vi "procesSiMAGE.vi"(0 "Cam Cluster out":T6={"incident ANGLE COMPENSATION"=[], "field of view /pixel"=0.0, "dp/B [MeV/C/B]"=[], "charge compensation"=[], "Momentum [MeV/C]"=[], "B [T]"=1.0, "energyDependence Input"=[], "pixel angle (y)"=[], "dp [MeV/C/] "=[], "angle 2Dfor spectrumj"=[], "dp [MeV/C] 2D"=[], "charge compensation 2D"=[], "Screen&Camera 2"={"Screen Orientation"="Regular", "Screen angle"="Flat", "Lens"=enum."FL1-f8x08", "Calibration (mm/pix)"=1.0}, "ROI info"={"npix-X"=0, "npix-Y"=0, "Left [pix]"=0.0, "Top [pix]"=0.0}, "Y 2D full angle"=[]}, 1 "Image":T2, 2 "empty image":bool, 5 "CamSettings.Cam 0":T3={"position"=0.0, "Field of view"=0.0, "start"=0.0, "end"=0.0, "center"=0.0, "Lens"=enum."FL1-f8x08", "Forward"=enum."off", "Spec_Calib_file 2"=path "Y:/100TWdata/ESMCalib/datFwd.txt", "map"=path "Y:/100TWdata/ESMCalib/mapFwd.txt", "y size"=0}, 12 "B [T]":dbl) -> (4 "Cam Cluster out 2":T6={"incident ANGLE COMPENSATION"=[], "field of view /pixel"=0.0, "dp/B [MeV/C/B]"=[], "charge compensation"=[], "Momentum [MeV/C]"=[], "B [T]"=1.0, "energyDependence Input"=[], "pixel angle (y)"=[], "dp [MeV/C/] "=[], "angle 2Dfor spectrumj"=[], "dp [MeV/C] 2D"=[], "charge compensation 2D"=[], "Screen&Camera 2"={"Screen Orientation"="Regular", "Screen angle"="Flat", "Lens"=enum."FL1-f8x08", "Calibration (mm/pix)"=1.0}, "ROI info"={"npix-X"=0, "npix-Y"=0, "Left [pix]"=0.0, "Top [pix]"=0.0}, "Y 2D full angle"=[]}, 6 "Sum Y":cluster{"Ramp Pattern":dbl[], dbl[]}, 8 "spec cluster":cluster{"dp [MeV/C]":dbl[], dbl[]}(graph), 10 "z":dbl[][](array[numeric]), 14 "time":u32)   [LabVIEW 2011]
uses:
  calib_Sub_Typdef.ctl
  ScreenCam2_TypDEf.ctl
  CamAndObj_TypDEf.ctl
  ROIInfo_TypDef.ctl
  CamSettingSUB_TypDEf.ctl
  OnOffTypeDef.ctl
  IMAQ Image.ctl
panel:
  out "x*y":dbl[][](array[numeric])
  out "time 2":u32
  out "spec cluster 2":T1(graph)
  out "Momentum [MeV/C]":dbl[](array[numeric])
  out "Boolean":bool
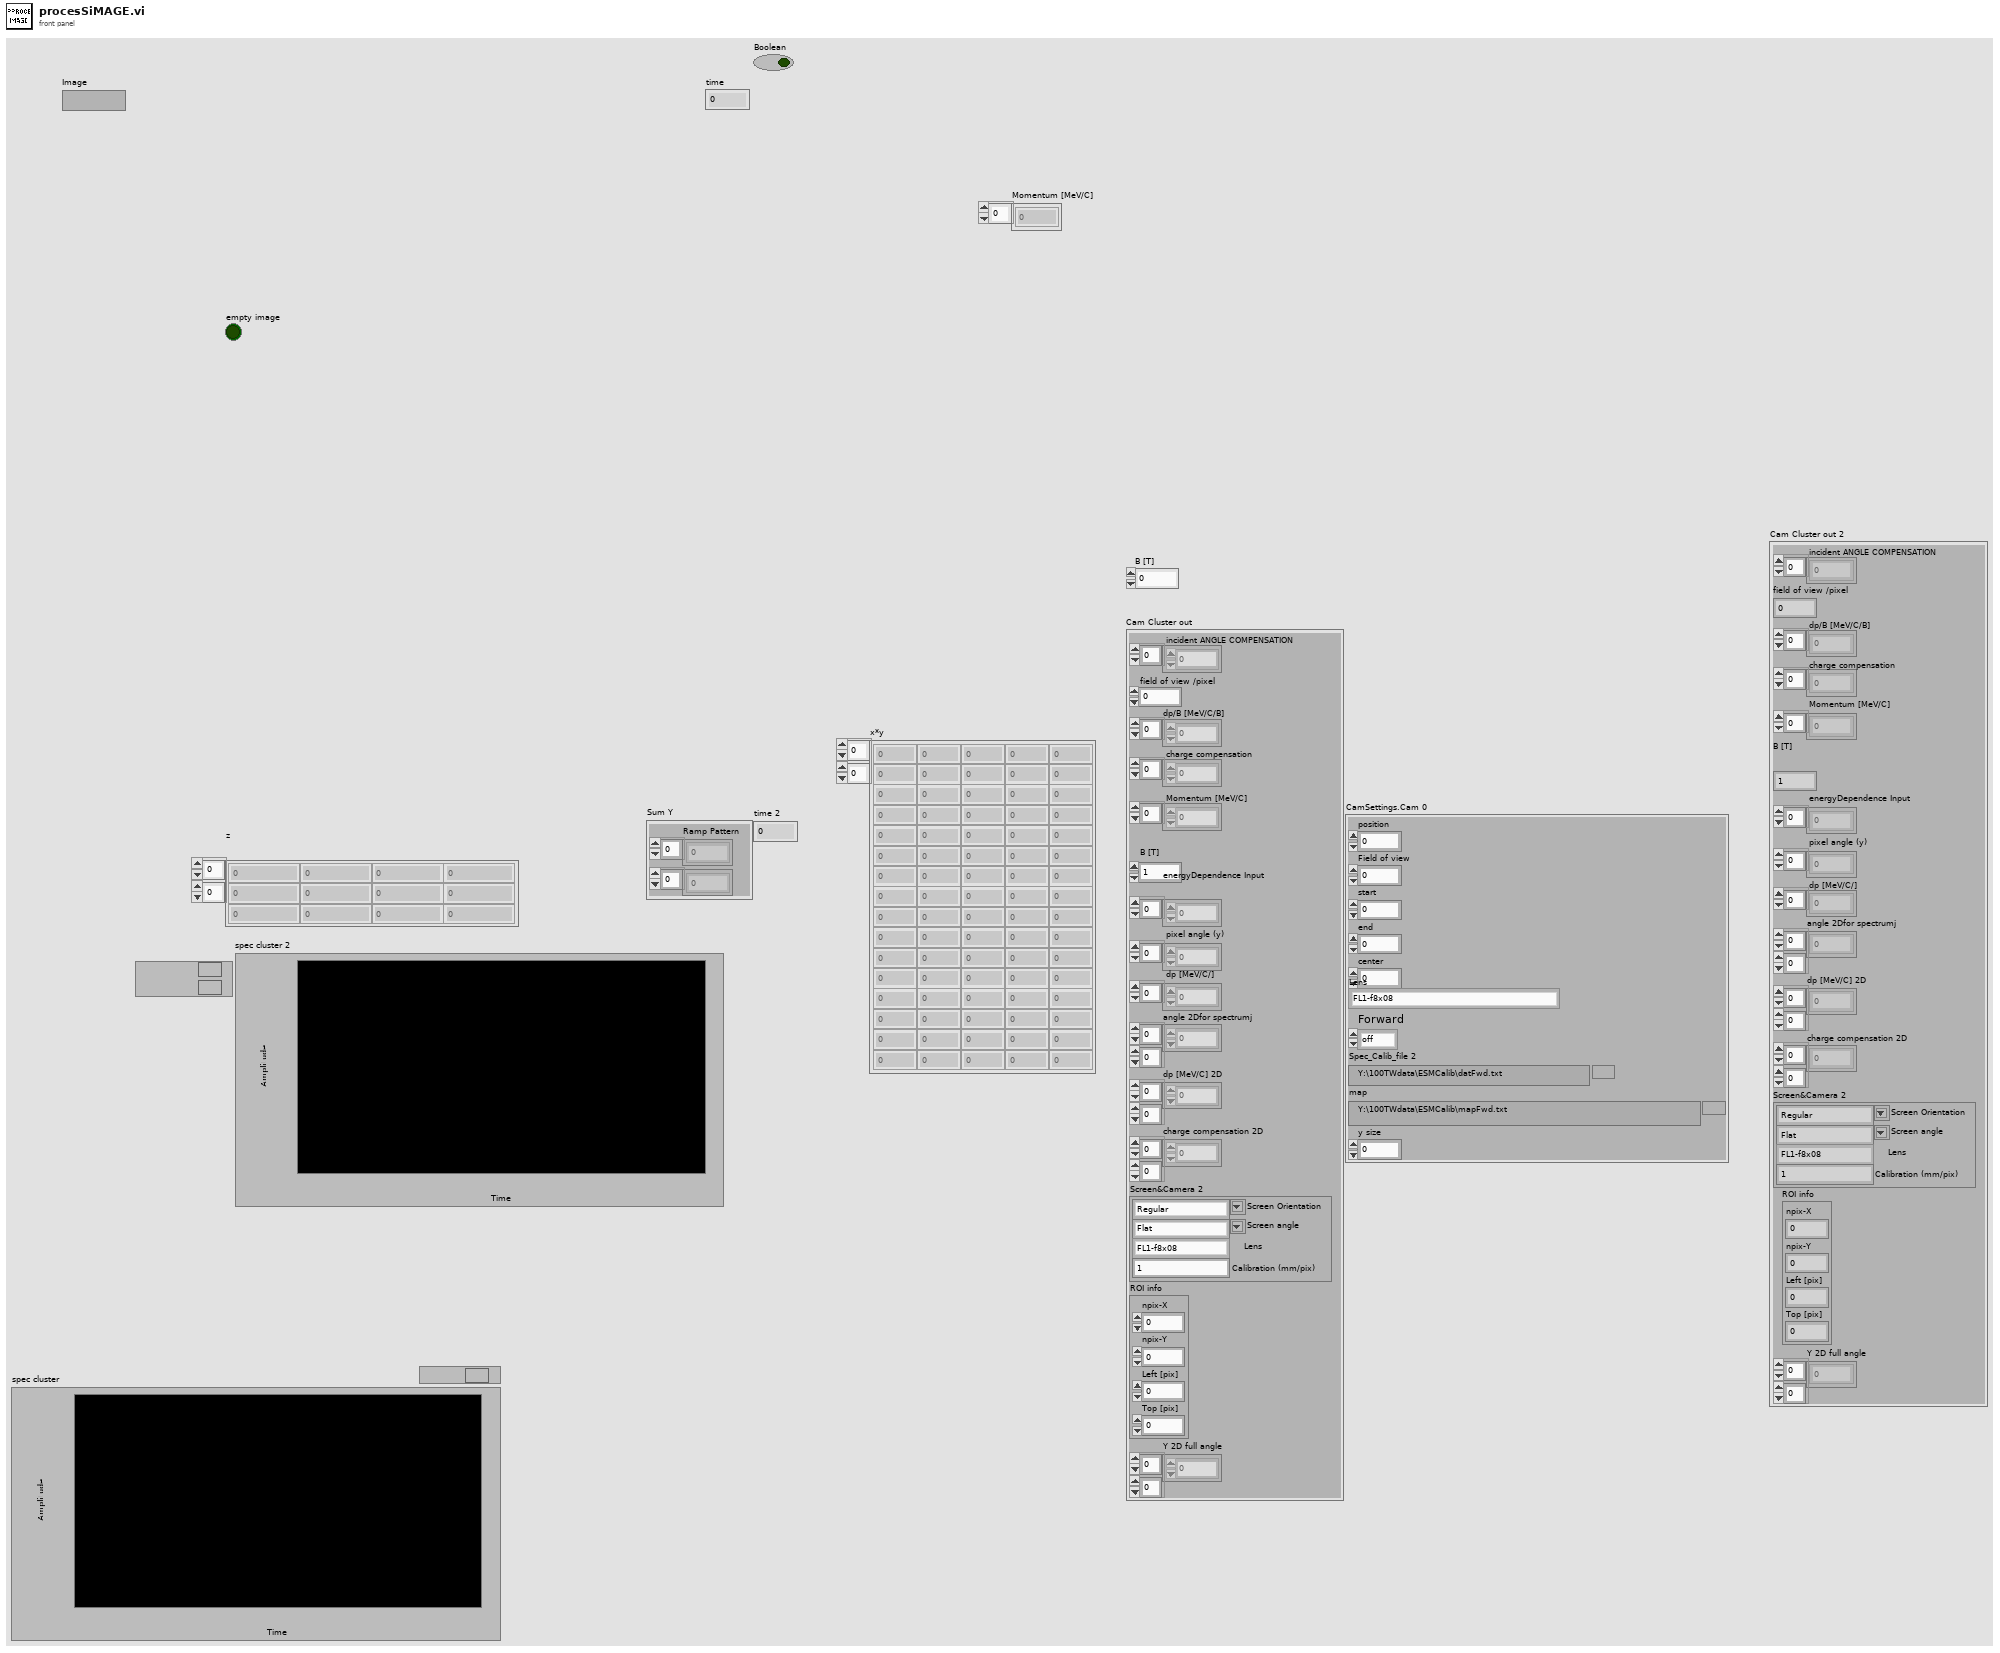
[diagram p1: front panel]
types:
  T1 = cluster{"Momentum [MeV/C]":dbl[], "Sum X (spectra)":dbl[]}[]
  T2 = typedef "IMAQ Image.ctl" = refnum<image>
  T3 = typedef "CamSettingSUB_TypDEf.ctl" = cluster{"position":dbl, "Field of view":dbl, "start":dbl, "end":dbl, "center":dbl, "Lens":T4, "Forward":T5, "Spec_Calib_file 2":path, "map":path, "y size":i32}
  T4 = typedef "CamAndObj_TypDEf.ctl" = enum16{"FL1-f8x08", "FL1-f8x06", "FL1-f8", "ch300-f50", "FL2G-f8", "FL3M14-f8", "FL3M14-f8x08", "FL3M14-f8x08(2x2)"}
  T5 = typedef "OnOffTypeDef.ctl" = enum16{"off", "on"}
  T6 = typedef "calib_Sub_Typdef.ctl" = cluster{"incident ANGLE COMPENSATION":dbl[], "field of view /pixel":dbl, "dp/B [MeV/C/B]":dbl[], "charge compensation":dbl[], "Momentum [MeV/C]":dbl[], "B [T]":dbl, "energyDependence Input":dbl[], "pixel angle (y)":dbl[], "dp [MeV/C/] ":dbl[], "angle 2Dfor spectrumj":dbl[][], "dp [MeV/C] 2D":dbl[][], "charge compensation 2D":dbl[][], "Screen&Camera 2":T7, "ROI info":T8, "Y 2D full angle":dbl[][]}
  T7 = typedef "ScreenCam2_TypDEf.ctl" = cluster{"Screen Orientation":string, "Screen angle":string, "Lens":T4, "Calibration (mm/pix)":dbl}
  T8 = typedef "ROIInfo_TypDef.ctl" = cluster{"npix-X":i32, "npix-Y":i32, "Left [pix]":dbl, "Top [pix]":dbl}
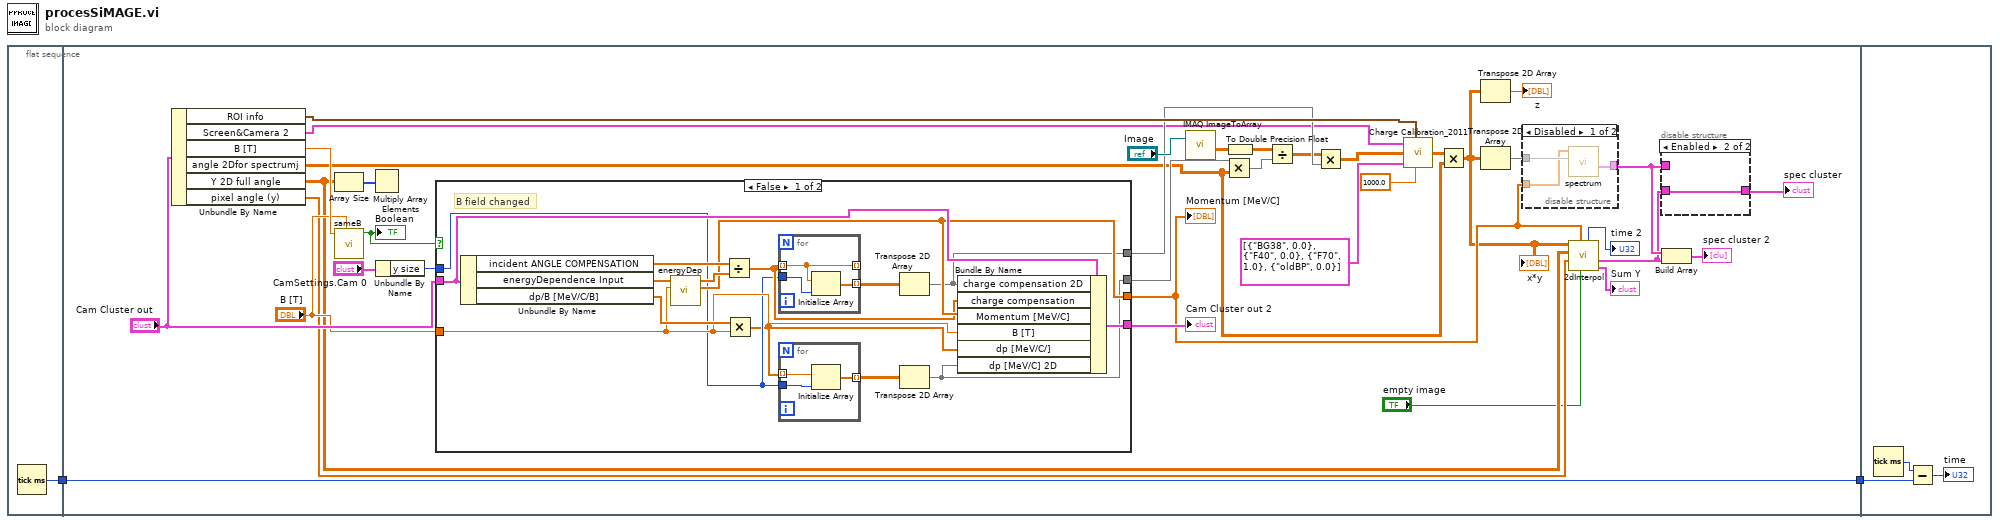
[diagram p0: block diagram]
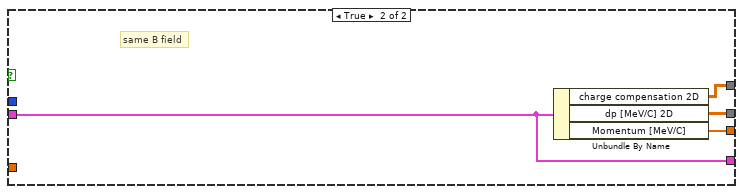
[diagram p4: hidden frame]
diagram:
  n1 = flat-sequence {
    tunnel: [w3] -> w1
    tunnel: [w32] -> w2
    tunnel: w1 -> [w32]
    tunnel: w2 -> [w71]
    frame #0 {
      n2 = Tick Count (ms)() -> (millisecond timer value=w3:u32)
    }
    frame #1 {
      n3 = Unbundle By Name("Cam Cluster out") -> ("ROI info"=w30:T8, "Screen&Camera 2"=w4:T7, "B [T]"=w39:dbl, "angle 2Dfor spectrumj"=w11:dbl[][], "Y 2D full angle"=w21:dbl[][], "pixel angle (y)"=w18:dbl[])
      n4 = Array Size(array=w21) -> (size(s)=w26:i32[])
      n5 = call "sameB.vi"("B [T] new"="B [T]", "B [T] old"=w39) -> ("Boolean"=w38:bool)  [unwired: 9 in]
      "Boolean" <- w38
      n6 = Multiply Array Elements(1:w26) -> ()  [unwired: 1 out]
      n7 = Unbundle By Name("CamSettings.Cam 0") -> ("y size"=w25:i32)
      n8 = case shown="False" w38 {
        tunnel: [w46 w69] -> w22
        tunnel: [w50 w68] -> w23
        tunnel: "Cam Cluster out" -> [w56 w67]
        tunnel: "B [T]" -> [w54 _]
        tunnel: [w53 w67] -> w36
        tunnel: [w52 w66] -> w20
        tunnel: w25 -> [w47 _]
        frame False {
          # "B field changed"
          n9 = Unbundle By Name(w56) -> ("incident ANGLE COMPENSATION"=w58:dbl[], "energyDependence Input"=w59:dbl[], "dp/B [MeV/C/B]"=w55:dbl[])
          n10 = call "energyDep.vi"("B [T]"=w54, "energy Dep in"=w59) -> ("Momentum [MeV/C]"=w52:dbl[], "energy dependence"=w57:dbl[])  [unwired: 8 in]
          n11 = Divide(x=w58, y=w57) -> (x/y=w48:dbl[])
          n12 = Multiply(x=w55, y=w54) -> (x*y=w45:dbl[])
          n13 = for {
            tunnel: [w60] -> _ mode=indexing
            tunnel: [w62] -> w49 mode=indexing
            tunnel: w47 -> [w61]
            tunnel: w48 -> [w60] mode=indexing
            n14 = Initialize Array(w60, w61) -> (w62:dbl[])
          }
          n15 = for {
            tunnel: w45 -> [w65] mode=indexing
            tunnel: [w64] -> w51 mode=indexing
            tunnel: w47 -> [w63]
            n16 = Initialize Array(w65, w63) -> (w64:dbl[])
          }
          n17 = Transpose 2D Array(2D array=w49) -> (transposed array=w46:dbl[][])
          n18 = Transpose 2D Array(2D array=w51) -> (transposed array=w50:dbl[][])
          n19 = Bundle By Name(cluster=w56, "charge compensation 2D"=w46, "charge compensation"=w48, "Momentum [MeV/C]"=w52, "B [T]"=w54, "dp [MeV/C/]"=w45, "dp [MeV/C] 2D"=w50) -> (w53:T6)
        }
        frame True {
          # "same B field"
          n20 = Unbundle By Name(w67) -> ("charge compensation 2D"=w69:dbl[][], "dp [MeV/C] 2D"=w68:dbl[][], "Momentum [MeV/C]"=w66:dbl[])
        }
      }
      "Cam Cluster out 2" <- w36
      "Momentum [MeV/C]" <- w20
      n21 = call "IMAQ ImageToArray"("Image"="Image") -> ("Image Pixels (Float)"=w8:sgl[][])  [unwired: 3 in, 4 out]
      n22 = Multiply(x=w23, y=w11) -> (x*y=w29:dbl[][])
      n23 = To Double Precision Float(number=w8) -> (double precision float=w7:dbl[][])
      n24 = Divide(x=w7, y=w29) -> (x/y=w14:dbl[][])
      n25 = Multiply(x=w14, y=w22) -> (x*y=w6:dbl[][])
      n26 = call "Charge Calibration_2011.vi"("Screen&Camera 2"=w4, "ROI infos"=w30, "Image (Counts)"=w6, "Filters"=cluster{"Name":string, "#Filters":dbl}[] [{"Name"="BG38", "#Filters"=0.0}, {"Name"="F40", "#Filters"=0.0}, {"Name"="F70", "#Filters"=1.0}, {"Name"="oldBP", "#Filters"=0.0}], "Electron energy (MeV)"=1000.0) -> ("Image (pC)"=w13:dbl[][])  [unwired: 4 in]
      n27 = Multiply(x=w13, y=w11) -> (x*y=w12:dbl[][])
      "x*y" <- w12
      n28 = Transpose 2D Array(2D array=w12) -> (transposed array=→"z":dbl[][])
      n29 = Transpose 2D Array(2D array=w12) -> (transposed array=w33:dbl[][])
      n30 = disable-structure shown="Disabled" {
        disable-tunnel: w33 -> [w42 _]
        disable-tunnel: w20 -> [w41 _]
        disable-tunnel: [w40 _] -> w17
        frame Disabled {
          n31 = call "spectrum.vi"("z in"=w42, "Momentum [MeV/C]"=w41) -> ("output cluster"=w40:cluster{"dp [MeV/C]":dbl[], dbl[]})  [unwired: 9 in]
        }
        frame Enabled {
        }
      }
      n32 = call "2dInterpol.vi"("empty image"="empty image", "Momentum [MeV/C]"=w20, "pixel angle (y)"=w18, "Y angles 2D"=w21, "Z"=w12) -> ("Sum Y"=→"Sum Y":cluster{"Ramp Pattern":dbl[], dbl[]}, "spec cluster 2"=w15:cluster{"Momentum [MeV/C]":dbl[], dbl[]}, "time: 2Dinter"=→"time 2":u32)  [unwired: 4 in]
      n33 = disable-structure shown="Enabled" {
        disable-tunnel: w17 -> [w43 _]
        disable-tunnel: [w43 w44] -> w16
        disable-tunnel: w15 -> [_ w44]
        frame Disabled {
        }
        frame Enabled {
        }
      }
      "spec cluster" <- w16
      n34 = Build Array(w17, w15) -> (→"spec cluster 2":cluster{"Momentum [MeV/C]":dbl[], dbl[]}[])
    }
    frame #2 {
      n35 = Tick Count (ms)() -> (millisecond timer value=w72:u32)
      n36 = Subtract(x=w72, y=w71) -> (x-y=→"time":u32)
    }
  }
